vi "SelectedGlobal.vi"(6 "cmd(Get)":enum16{"Get", "Set"}(ring), 8 "error in (no error)":errorcluster, 11 "selected in":bool) -> (0 "error out":errorcluster, 3 "selected out out":bool)   [LabVIEW 2009]
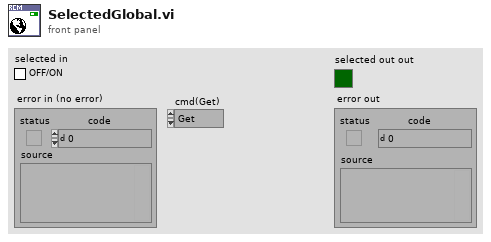
[diagram p1: front panel]
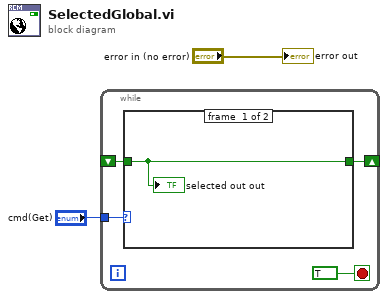
[diagram p0: block diagram]
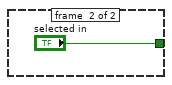
[diagram p2: hidden frame]
diagram:
  n1 = while {
    tunnel: "cmd(Get)" -> [w5]
    shift-right: [w4] -> _
    shift-left: _ -> [w3]
    stop <- TRUE stop-if-true
    n2 = case shown="\"Set\"" w5 {
      tunnel: [w7 "selected in"] -> w4
      tunnel: w3 -> [w7 _]
      frame #0 {
        "selected out out" <- w7
      }
      frame #1 {
      }
    }
  }
  "error out" <- "error in (no error)"
